vi "SerialTx.vi"(1 "SerialSettings":T1={"SerialPort"="RS232\\Port1", "TxFIFO"="U64FIFOTx", "RxFIFO"="U64FIFORx", "TimestampRegister"="TimestampRegister"}) -> ()   [LabVIEW 2016, in "FPGASerial.lvlib"]
uses:
  FPGASerial.lvlib
  DataTypes/SerialSettings.ctl
  <vilib>/rvi/Emulation/niFpgaGetClockAttributes.vi
  <vilib>/rvi/Emulation/niFpgaSctlEmulationGetInTimedLoop.vi
  <vilib>/rvi/Emulation/niFpgaEmulationReportErrorSimple.vi
  <vilib>/rvi/DataTransferAndStorage/Container/Common/niFpgaContainerExecOnDevCompGetState.vi
  <vilib>/rvi/Emulation/niFpgaEmulationIsFPGAContextNoSignature.vi
  <vilib>/rvi/errors/niFpgaSetErrorForExecOnDevCompSimple.vi
  <vilib>/rvi/eio/common/nirviEmuReportErrorAndStop.vi
  <vilib>/rvi/DataTransferAndStorage/Container/Common/niFpgaContainerGetUniqueNameForEmu.vi
  <vilib>/rvi/FIFO/Fifo_Resource/nirvififoEmulationSetSize.vi
  <vilib>/rvi/FIFO/Fifo_Resource/nirviFifoEmulationQueueMgr.vi
  <instcachedir>/0/nirviFifoEmulationQueueMgr_E5CAEC123FF24DC58D834DCA3CDAA9B5.lvgen/nirviFifoEmulationQueueMgr_E5CAEC123FF24DC58D834DCA3CDAA9B5_007.vi
  <vilib>/rvi/FIFO/Fifo_Resource/nirvififoEmulationDetermineInputValidOut.vi
  <vilib>/rvi/FIFO/Fifo_Resource/nirvififoEmulationCreateLock.vi
  <vilib>/rvi/Emulation/niFpgaProcessEmulError.vi
  <vilib>/rvi/FIFO/Fifo_Resource/nirvififoEmulationObtainLock.vi
  <vilib>/rvi/FIFO/Fifo_Resource/nirvififoEmulationReleaseLock.vi
  <vilib>/rvi/occurrence/nirviWaitOnOccurrenceBase.vi
  <vilib>/rvi/errors/nirviReportUnexpectedCaseInternalError.vi
  <vilib>/rvi/errors/nirviReportUnexpectedCaseInternalError (U32).vi
  <vilib>/Utility/error.llb/Clear Errors.vi
  <vilib>/rvi/interface/RandomDataEmulation/niFpgaRandomDataHandleErrors.vi
  <vilib>/rvi/eio/common/nirviEmuTemplateMethod_errors.vi
  <vilib>/rvi/Emulation/niFpgaCriticalErrorInLSC.vi
  <vilib>/rvi/DataTransferAndStorage/Container/XNode/niFpgaContainer.xnode
  <vilib>/rvi/FIFO/Fifo_Resource/niFpgaFifoEmulationRefIn.vi
  <vilib>/eio/EIOMethodNode/EIOMethodNode.xnode
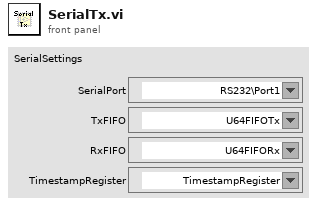
[diagram p1: front panel]
types:
  T1 = typedef "FPGASerial.lvlib/SerialSettings.ctl" = cluster{"SerialPort":refnum<k21>, "TxFIFO":refnum<k21>, "RxFIFO":refnum<k21>, "TimestampRegister":refnum<k21>}
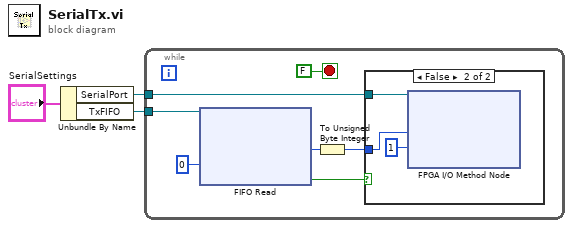
[diagram p0: block diagram]
diagram:
  n1 = Unbundle By Name("SerialSettings") -> ("SerialPort"=w2:refnum<k21>, "TxFIFO"=w3:refnum<k21>)
  n2 = while {
    tunnel: w3 -> [w10]
    tunnel: w2 -> [w9]
    stop <- FALSE stop-if-true
    n3 = xnode "FIFO Read"("Timeout"=0, "FIFO In"=w10) -> ("Element"=w4:u64, "Timed Out?"=w6:bool)  [unwired: 1 out]
    n4 = To Unsigned Byte Integer(number=w4) -> (unsigned 8bit integer=w5:u8)
    n5 = case shown="False" w6 {
      tunnel: w9 -> [_ w13]
      tunnel: w5 -> [_ w12]
      frame True {
      }
      frame False {
        n6 = xnode "FPGA I/O Method Node"("FPGA I/O In"=w13, "Data"=w12, "Timeout (ms)"=1) -> ()  [unwired: 2 out]
      }
    }
  }
